vi "Uninitialize.vi"(8 "error in (no error)":errorcluster) -> (0 "error out":errorcluster)   [LabVIEW 2015, in "lvwpcap.lvlib"]
doc: "This VI uninitializes the packet sniffer utility."
uses:
  lvwpcap.lvlib
  LVpcap.dll
panel:
  # "Select Help»Show Context Help and move the cursor over the VI icon to display help for this VI."
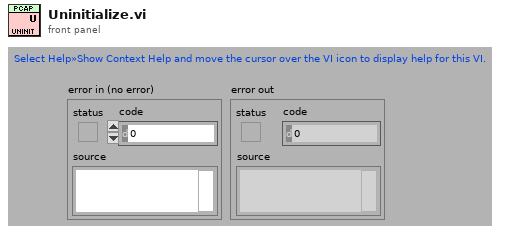
[diagram p1: front panel]
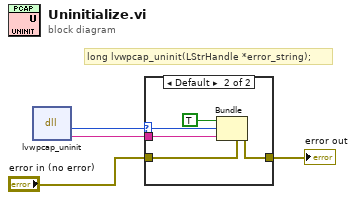
[diagram p0: block diagram]
diagram:
  # "long lvwpcap_uninit(LStrHandle *error_string);"
  n1 = dll-call lib="C:/Users/plc/Desktop/WPCAP/Lib/LVpcap.dll" fn="lvwpcap_uninit"() -> ("return type"=w4:i32, "error_string"=w3:string)  [unwired: 4 in, 2 out]
  n2 = case shown="Default" w4 {
    selector: w4 -> [_ w9]
    tunnel: w3 -> [_ w8]
    tunnel: "error in (no error)" -> [w5 w10]
    tunnel: [w5 w6] -> w1
    frame 0 {
    }
    frame Default {
      n3 = Bundle(cluster=w10, "status"=TRUE, "code"=w9, "source"=w8) -> (w6:errorcluster)
    }
  }
  "error out" <- w1
